vi "StringArray step.vi"(11 "NUOVO STEP":T1 {"Tempo Step[s]" format="%#.1f"}) -> (3 "Array":string[](array[string]))   [LabVIEW 2019]
uses:
  controls/STEP.ctl
  controls/Caratteristiche step.ctl
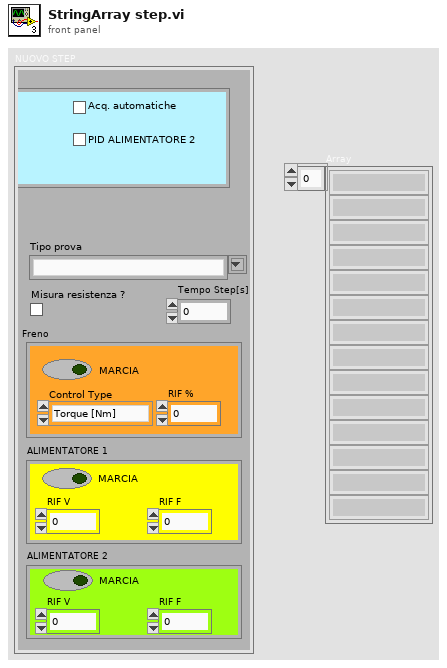
[diagram p1: front panel]
types:
  T1 = typedef "STEP.ctl" = cluster{"Tipo prova":string, "Misura resistenza ?":bool, "Tempo Step[s]":dbl, "Freno":cluster{"MARCIA":bool, "Control Type":enum32{"Torque [Nm]", "Power [W]", "Speed [RPM]", "Corrente [A]"}, "RIF %":dbl}, "ALIMENTATORE 1":cluster{"MARCIA":bool, "RIF V":dbl, "RIF F":dbl}, "ALIMENTATORE 2":cluster{"MARCIA":bool, "RIF V":dbl, "RIF F":dbl}, "Caratteristiche step":T2}
  T2 = typedef "Caratteristiche step.ctl" = cluster{"Attendi stabilizz.":bool, "Acq. fine step?":bool, "Acq. automatiche":bool, "PID FRENO":bool, "PID ALIMENTATORE 1":bool, "PID ALIMENTATORE 2":bool, "CAMBIA PROVA SE EQ. TERMICO":bool}
  T3 = enum32{"Torque [Nm]", "Power [W]", "Speed [RPM]", "Corrente [A]"}
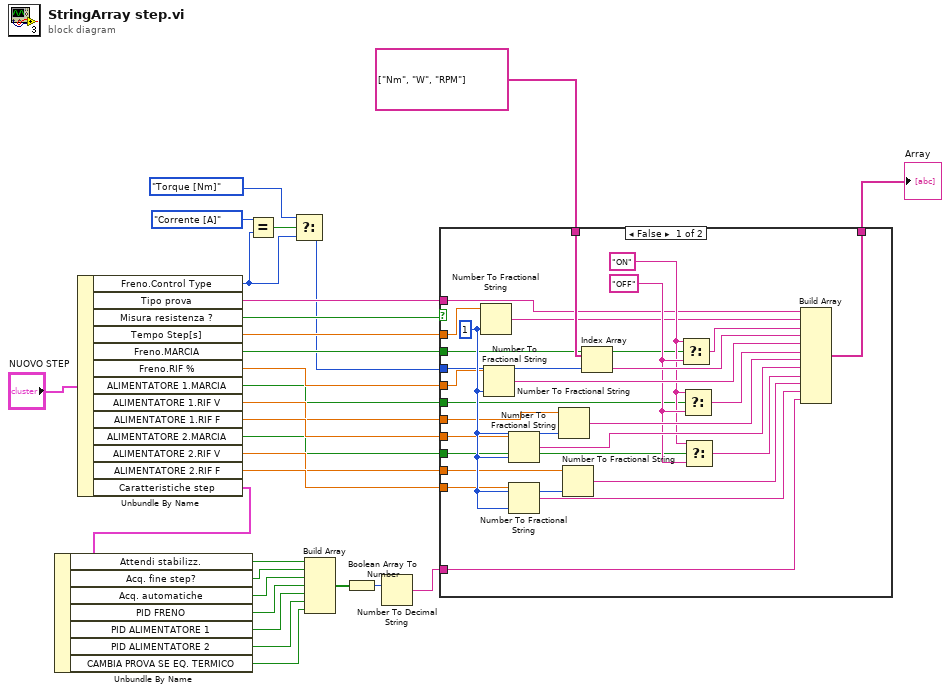
[diagram p0: block diagram]
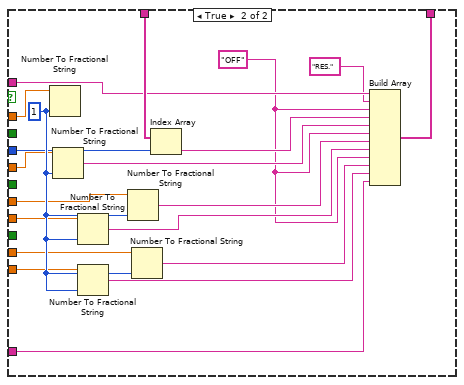
[diagram p2: hidden frame]
diagram:
  n1 = Unbundle By Name("NUOVO STEP") -> ("Freno.Control Type"=w3:T3, "Tipo prova"=w18:string, "Misura resistenza ?"=w17:bool, "Tempo Step[s]"=w23:dbl, "Freno.MARCIA"=w19:bool, "Freno.RIF %"=w24:dbl, "ALIMENTATORE 1.MARCIA"=w20:bool, "ALIMENTATORE 1.RIF V"=w25:dbl, "ALIMENTATORE 1.RIF F"=w26:dbl, "ALIMENTATORE 2.MARCIA"=w21:bool, "ALIMENTATORE 2.RIF V"=w27:dbl, "ALIMENTATORE 2.RIF F"=w28:dbl, "Caratteristiche step"=w16:T2)
  n2 = Unbundle By Name(w16) -> ("Attendi stabilizz."=w15:bool, "Acq. fine step?"=w14:bool, "Acq. automatiche"=w13:bool, "PID FRENO"=w12:bool, "PID ALIMENTATORE 1"=w11:bool, "PID ALIMENTATORE 2"=w10:bool, "CAMBIA PROVA SE EQ. TERMICO"=w9:bool)
  n3 = Equal?(x=T3."Corrente [A]" ("Freno.Control Type"), y=w3) -> (x = y?=w5:bool)
  n4 = Select(t=T3."Torque [Nm]" ("Freno.Control Type"), s=w5, f=w3) -> (s? t:f=w2:T3)
  n5 = Build Array(w15, w14, w13, w12, w11, w10, w9) -> (w8:bool[])
  n6 = Boolean Array To Number(Boolean array=w8) -> (number=w7:u32)
  n7 = Number To Decimal String(number=w7) -> (decimal integer string=w6:string)  [unwired: 1 in]
  n8 = case shown="False" w17 {
    tunnel: [w57 w77] -> w30
    tunnel: w28 -> [w46 w69]
    tunnel: w27 -> [w45 w68]
    tunnel: w26 -> [w44 w67]
    tunnel: w25 -> [w43 w66]
    tunnel: w24 -> [w42 w65]
    tunnel: w23 -> [w41 w64]
    tunnel: w2 -> [w40 w63]
    tunnel: string[] ["Nm", "W", "RPM"] -> [w39 w62]
    tunnel: w21 -> [w36 _]
    tunnel: w20 -> [w35 _]
    tunnel: w19 -> [w34 _]
    tunnel: w18 -> [w33 w61]
    tunnel: w6 -> [w32 w60]
    frame False {
      w54 = i16 1 ("precision (6)")
      w38 = "OFF"
      w37 = "ON"
      n9 = Number To Fractional String(number=w41, precision (6)=w54) -> (F-format string=w31:string)  [unwired: 2 in]
      n10 = Number To Fractional String(number=w42, precision (6)=w54) -> (F-format string=w47:string)  [unwired: 2 in]
      n11 = Number To Fractional String(number=w44, precision (6)=w54) -> (F-format string=w50:string)  [unwired: 2 in]
      n12 = Number To Fractional String(number=w46, precision (6)=w54) -> (F-format string=w53:string)  [unwired: 2 in]
      n13 = Number To Fractional String(number=w43, precision (6)=w54) -> (F-format string=w49:string)  [unwired: 2 in]
      n14 = Number To Fractional String(number=w45, precision (6)=w54) -> (F-format string=w52:string)  [unwired: 2 in]
      n15 = Index Array(array=w39, index=w40) -> (element=w56:string)
      n16 = Select(t=w37, s=w34, f=w38) -> (s? t:f=w55:string)
      n17 = Select(t=w37, s=w35, f=w38) -> (s? t:f=w48:string)
      n18 = Select(t=w37, s=w36, f=w38) -> (s? t:f=w51:string)
      n19 = Build Array(w33, w31, w55, w56, w47, w48, w49, w50, w51, w52, w53, w32) -> (w57:string[])
    }
    frame True {
      w75 = i16 1 ("precision (6)")
      w59 = "OFF"
      n20 = Number To Fractional String(number=w64, precision (6)=w75) -> ()  [unwired: 2 in, 1 out]
      n21 = Number To Fractional String(number=w65, precision (6)=w75) -> (F-format string=w70:string)  [unwired: 2 in]
      n22 = Number To Fractional String(number=w67, precision (6)=w75) -> (F-format string=w72:string)  [unwired: 2 in]
      n23 = Number To Fractional String(number=w69, precision (6)=w75) -> (F-format string=w74:string)  [unwired: 2 in]
      n24 = Number To Fractional String(number=w66, precision (6)=w75) -> (F-format string=w71:string)  [unwired: 2 in]
      n25 = Number To Fractional String(number=w68, precision (6)=w75) -> (F-format string=w73:string)  [unwired: 2 in]
      n26 = Index Array(array=w62, index=w63) -> (element=w76:string)
      n27 = Build Array(w61, "RES." ("element"), w59, w76, w70, w59, w71, w72, w59, w73, w74, w60) -> (w77:string[])
    }
  }
  "Array" <- w30
